vi "JSON_sandbox.vi"() -> ()   [LabVIEW 2013]
panel:
  out "value":cluster{"Array":dbl[], "number":dbl}
  in  "String":string
  out "JSON string":string
  in  "Cluster":cluster{"Array":dbl[], "number":i32}
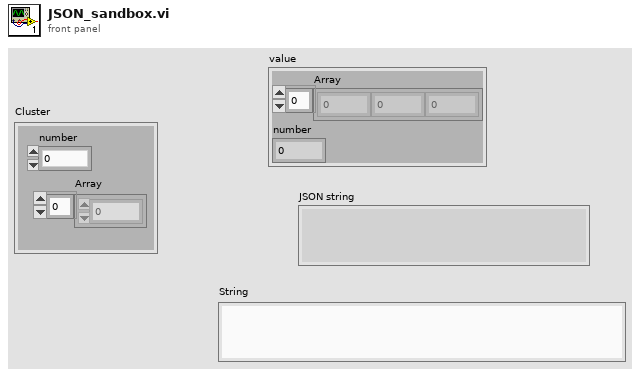
[diagram p1: front panel]
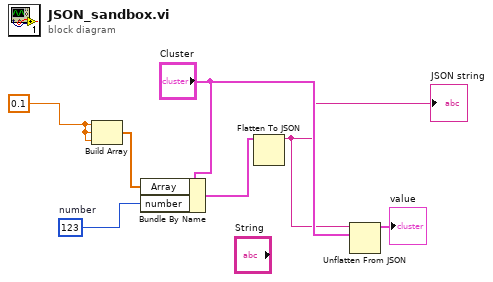
[diagram p0: block diagram]
diagram:
  w6 = 123  # number
  w7 = 0.1 ("element")
  n1 = Build Array(w7, w7, w7) -> (w3:dbl[])
  n2 = Bundle By Name(cluster="Cluster", "Array"=w3, "number"=w6) -> (w5:cluster{"Array":dbl[], "number":i32})
  n3 = Flatten To JSON(anything=w5) -> (JSON string=w1:string)  [unwired: 2 in, 1 out]
  "JSON string" <- w1
  n4 = Unflatten From JSON(JSON string=w1, type and defaults="Cluster") -> (value=→"value":cluster{"Array":dbl[], "number":i32})  [unwired: 5 in, 1 out]
